vi "PLL_On_Off (SubVI_NH).vi"(8 "error in (no error)":errorcluster, 9 "Output ON/OFF (F=OFF)":bool, 10 "delay":dbl=1.0 format="%#_3p", 11 "Application in":refnum<vi>) -> (0 "error out":errorcluster, 3 "Application out":refnum<vi>)   [LabVIEW 2014]
uses:
  <userlib>/Nanonis Prog Interface V5/Nanonis Prog Interface.lvlib
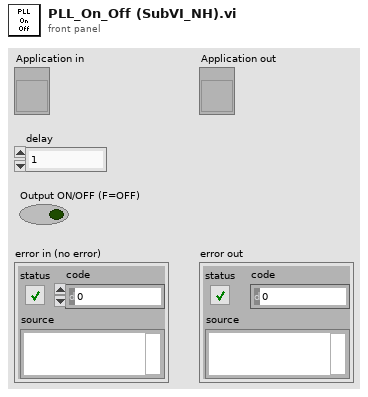
[diagram p1: front panel]
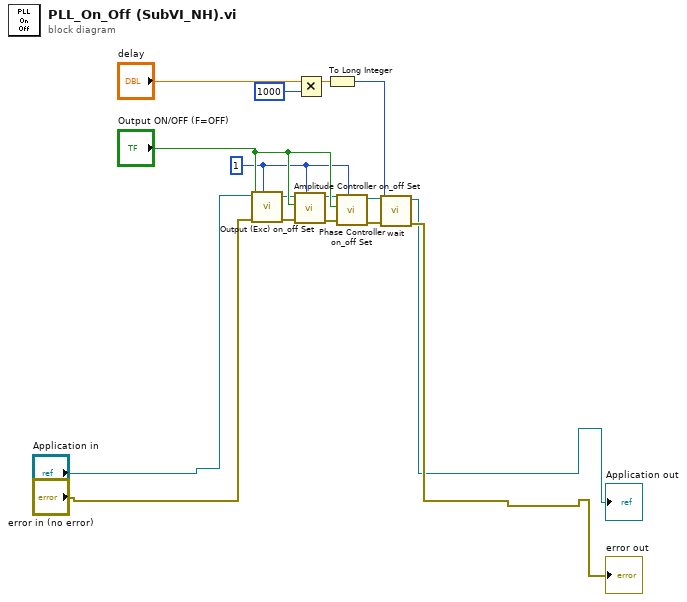
[diagram p0: block diagram]
diagram:
  w8 = 1 ("Modulator index")
  n1 = call <userlib>:"Output (Exc) on_off Set.vi"("Modulator index"=w8, "Error in (no error)"="error in (no error)", "Output ON/OFF (F=OFF)"="Output ON/OFF (F=OFF)", "Application ref in"="Application in") -> ("Error out"=w5:errorcluster, "Application ref out"=w4:refnum<vi>)  [unwired: 6 in]
  n2 = call <userlib>:"Amplitude Controller on_off Set.vi"("Modulator index"=w8, "Error in (no error)"=w5, "Amplitude controller ON/OFF"="Output ON/OFF (F=OFF)", "Application ref in"=w4) -> ("Error out"=w7:errorcluster, "Application ref out"=w6:refnum<vi>)  [unwired: 6 in]
  n3 = Multiply(x="delay", y=u32 1000) -> (x*y=w3:dbl)
  n4 = To Long Integer(number=w3) -> (32bit integer=w1:i32)
  n5 = call <userlib>:"Phase Controller on_off Set.vi"("Modulator index"=w8, "Error in (no error)"=w7, "Phase controller ON/OFF"="Output ON/OFF (F=OFF)", "Application ref in"=w6) -> ("Error out"=w11:errorcluster, "Application ref out"=w10:refnum<vi>)  [unwired: 6 in]
  n6 = call "wait.vi"("error in"=w11, "milliseconds to wait"=w1, "application reference in"=w10) -> ("error out"=→"error out":errorcluster, "application reference out"=→"Application out":refnum<vi>)  [unwired: 7 in]
